vi "Get All Ports.vi"(8 "error in":errorcluster, 11 "Ballard MIL-STD 1553 custom device in":T1 format="%.0x") -> (0 "error out":errorcluster, 2 "ports":T1[](array[typedef]) format="%.0x", 3 "Ballard MIL-STD 1553 custom device out":T1 format="%.0x")   [LabVIEW 2020, in "Ballard MIL-STD-1553 Scripting.lvlib"]
doc: "Returns references to all <b>ports</b> within the <b>Ballard MIL-STD-1553 custom device in</b>."
uses:
  Ballard MIL-STD-1553 Scripting.lvlib
  <vilib>/NI VeriStand/Custom Device API/Custom Device Item Ref.ctl
  Constants.vi
  <vilib>/NI VeriStand/Custom Device Tools/Custom Device Utility Library/NI VeriStand - Search for All Items by GUID.vi
  <vilib>/NI VeriStand/Custom Device Tools/Custom Device Utility Library/Custom Device Utility Library.lvlib
  <vilib>/NI VeriStand/Custom Device API/Custom Device API.lvlib
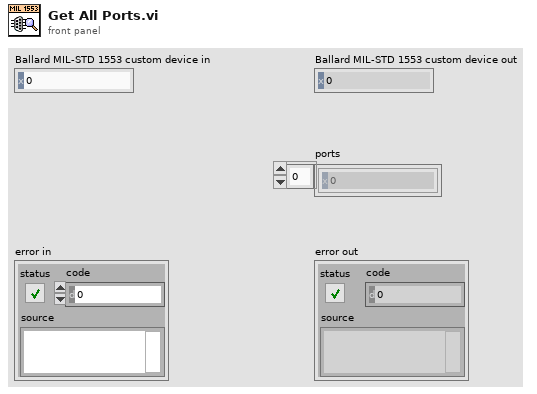
[diagram p1: front panel]
types:
  T1 = typedef "Custom Device API.lvlib/Custom Device Item Ref.ctl" = u64
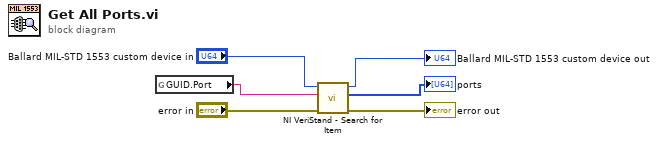
[diagram p0: block diagram]
diagram:
  n1 = global read "Constants.vi" "GUID.Port"() -> (w6:string)
  n2 = call-poly <vilib>:"NI VeriStand - Search for Item.vi"("error in"="error in", "Item GUID"=w6, "Section Ref in"="Ballard MIL-STD 1553 custom device in") -> ("error out"=→"error out":errorcluster, "Item Refs"=→"ports":T1[], "Section Ref out"=→"Ballard MIL-STD 1553 custom device out":T1)  [unwired: 5 in, 1 out]
